vi "Read Bit.vi"(8 "error in":errorcluster, 10 "PLC Bit Address":string="B3:0/0", 11 "IP Address:":string="192.168.100.15") -> (0 "error out":errorcluster, 3 "Result":bool)   [LabVIEW 2018]
uses:
  <vilib>/ethernetip/ethernetip.lvlib
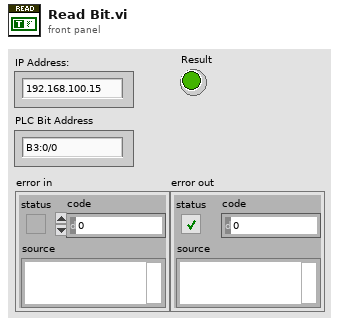
[diagram p1: front panel]
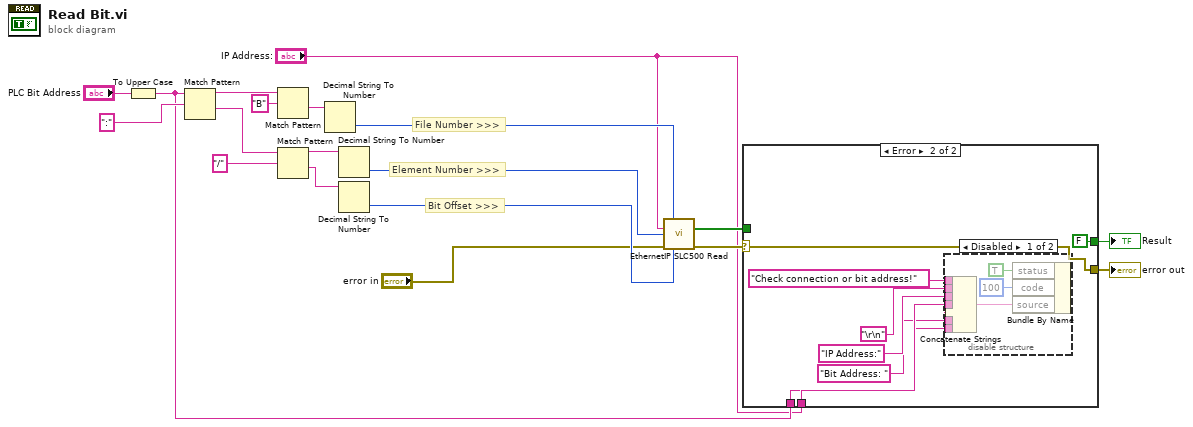
[diagram p0: block diagram]
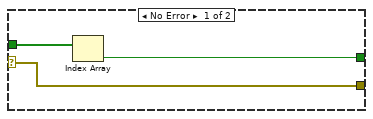
[diagram p2: hidden frame]
diagram:
  # "Bit Offset >>>"
  # "Element Number >>>"
  # "File Number >>>"
  n1 = To Upper Case(1:"PLC Bit Address") -> (0:w2:string)
  n2 = Match Pattern(string=w2, regular expression=":") -> (before substring=w18:string, after substring=w13:string)  [unwired: 1 in, 2 out]
  n3 = Match Pattern(string=w18, regular expression="B") -> (after substring=w15:string)  [unwired: 1 in, 3 out]
  n4 = Match Pattern(string=w13, regular expression="/") -> (before substring=w11:string, after substring=w9:string)  [unwired: 1 in, 2 out]
  n5 = Decimal String To Number(string=w15) -> (number=w14:i32)  [unwired: 2 in, 1 out]
  n6 = Decimal String To Number(string=w11) -> (number=w10:i32)  [unwired: 2 in, 1 out]
  n7 = Decimal String To Number(string=w9) -> (number=w8:i32)  [unwired: 2 in, 1 out]
  n8 = call-poly <vilib>:"EthernetIP SLC500 Read.vi"("File Number"=w14, "Network Path"="IP Address:", "Element Number"=w10, "error in"="error in", "Bit Offset"=w8) -> ("Data"=w5:bool[], "error out"=w6:errorcluster)  [unwired: 8 in, 1 out]
  n9 = case shown="Error" w6 {
    selector: w6 -> [w20 w23]
    tunnel: w5 -> [w22 _]
    tunnel: [w21 FALSE] -> w4
    tunnel: [w20 w23] -> w3
    tunnel: w2 -> [_ w24]
    tunnel: "IP Address:" -> [_ w27]
    frame No Error {
      n10 = Index Array(array=w22) -> (element=w21:bool)  [unwired: 1 in]
    }
    frame Error {
      n11 = disable-structure shown="Disabled" {
        disable-tunnel: "Check connection or bit address!" ("source") -> [w37 _]
        disable-tunnel: "IP Address:" -> [w36 _]
        disable-tunnel: w27 -> [w34 _]
        disable-tunnel: "\r\n" -> [w33 _]
        disable-tunnel: "Bit Address: " -> [w32 _]
        disable-tunnel: w24 -> [w31 _]
        frame Disabled {
          n12 = Concatenate Strings(w37, w33, w36, w34, w33, w32, w31) -> (w35:string)
          n13 = Bundle By Name("status"=TRUE, "code"=100, "source"=w35) -> ()  [unwired: 1 in, 1 out]
        }
        frame Enabled {
        }
      }
    }
  }
  "Result" <- w4
  "error out" <- w3
